vi "SwissSPAD Live_Save HDF5 8-bit Gate Image.vi"(4 "Compression Level (0-9)":u8=9 max=9, 6 "Compression":bool, 7 "Replace?":bool, 8 "error in (no error)":errorcluster, 9 "Image Name":string, 10 "Data":u8[][](array[numeric]), 11 "ref in":T1 format="%.0x") -> (0 "error out":errorcluster, 3 "ref out":T1 format="%.0x")   [LabVIEW 2021]
uses:
  <vilib>/addons/h5labview2/base/hid_t.ctl
  <vilib>/addons/h5labview2/base/lib_path.vi
  <vilib>/addons/h5labview2/base/H5Equery.vi
  <vilib>/addons/h5labview2/dataset/H5Dwrite.llb/H5Dwrite.xnode
  <vilib>/addons/h5labview2/props/H5P.lvlib
  <vilib>/addons/h5labview2/space/H5S.lvlib
  <vilib>/addons/h5labview2/type/H5T.lvlib
  <vilib>/addons/h5labview2/dataset/H5D.lvlib
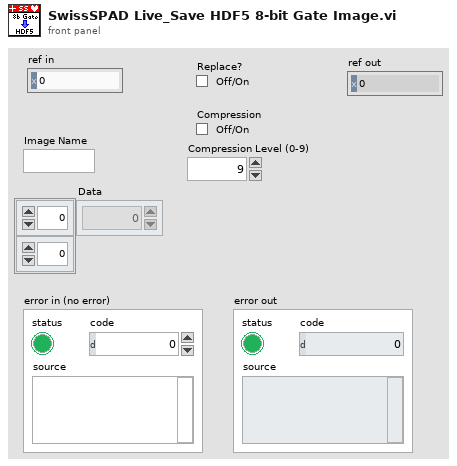
[diagram p1: front panel]
types:
  T1 = typedef "hid_t.ctl" = i32
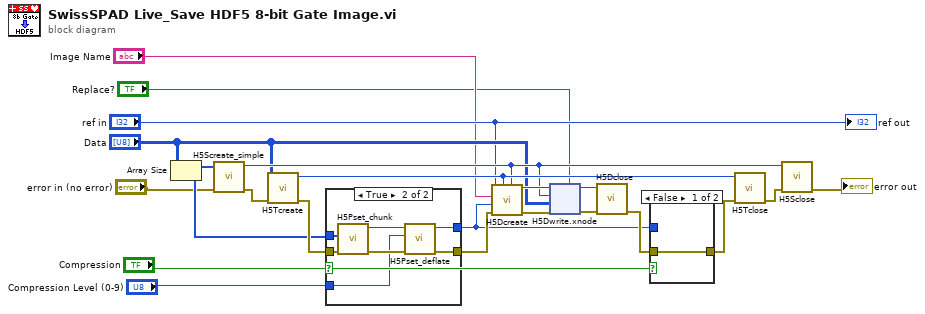
[diagram p0: block diagram]
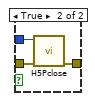
[diagram p2: hidden frame]
diagram:
  n1 = Array Size(array="Data") -> (size(s)=w10:i32[])
  n2 = call <vilib>:"H5Screate_simple.vi"("error in (no error)"="error in (no error)", "dims"=w10) -> ("error out"=w18:errorcluster, "space out"=w12:T1)  [unwired: 7 in, 1 out]
  n3 = call <vilib>:"H5Tcreate.vi"("error in (no error)"=w18, "type variant"="Data") -> ("error out"=w17:errorcluster, "type out"=w14:i32)  [unwired: 7 in, 1 out]
  n4 = case shown="True" "Compression" {
    tunnel: w17 -> [w23 w30]
    tunnel: [_ w29] -> w2
    tunnel: [w23 w26] -> w11
    tunnel: w10 -> [_ w25]
    tunnel: "Compression Level (0-9)" -> [_ w24]
    frame False {
    }
    frame True {
      n5 = call <vilib>:"H5Pset_chunk.vi"("error in (no error)"=w30, "chunk size"=w25) -> ("error out"=w27:errorcluster, "prop out"=w28:T1)  [unwired: 8 in]
      n6 = call <vilib>:"H5Pset_deflate.vi"("error in (no error)"=w27, "level"=w24, "prop in"=w28) -> ("error out"=w26:errorcluster, "prop out"=w29:T1)  [unwired: 7 in]
    }
  }
  n7 = call <vilib>:"H5Dcreate.vi"("space id"=w12, "type id"=w14, "error in (no error)"=w11, "props id"=w2, "name"="Image Name", "loc in"="ref in") -> ("error out"=w16:errorcluster, "dset out"=w19:T1)  [unwired: 2 in]
  n8 = xnode "H5Dwrite.xnode"("replace? (F)"="Replace?", "error in (no error)"=w16, "data"="Data", "file space"=w12, "ref in"=w19) -> ("error out"=w22:errorcluster, "ref out"=w20:i32)  [unwired: 2 in, 1 out]
  n9 = call <vilib>:"H5Dclose.vi"("error in (no error)"=w22, "dset in"=w20) -> ("error out"=w21:errorcluster)  [unwired: 9 in]
  n10 = case shown="False" "Compression" {
    tunnel: w21 -> [w31 w34]
    tunnel: [w31 w33] -> w15
    tunnel: w2 -> [_ w32]
    frame False {
    }
    frame True {
      n11 = call <vilib>:"H5Pclose.vi"("error in (no error)"=w34, "props in"=w32) -> ("error out"=w33:errorcluster)  [unwired: 9 in]
    }
  }
  n12 = call <vilib>:"H5Tclose.vi"("error in (no error)"=w15, "type in"=w14) -> ("error out"=w13:errorcluster)  [unwired: 9 in]
  n13 = call <vilib>:"H5Sclose.vi"("error in (no error)"=w13, "space in"=w12) -> ("error out"=→"error out":errorcluster)  [unwired: 9 in]
  "ref out" <- "ref in"
